vi "Get further extended drive and motor status.vi"(0 "COM port":refnum<visa-resource-name>, 7 "Drive address":T7=1 items=["0", "1", "2", "3", "4", "5", "6", "7", "8", "9", "10", "11", "12", "13", "14", "15", "16", "17", "18", "19", "20", "21", "22", "23", "24", "25", "26", "27", "28", "29", "30", "31", "32", "33", "34", "35", "36", "37", "38", "39", "40", "41", "42", "43", "44", "45", "46", "47", "48", "49", "50", "51", "52", "53", "54", "55", "56", "57", "58", "59", "60", "61", "62", "63"]) -> (4 "No errors":bool, 6 "Modbus error cluster":T1={"Checksum ok"=FALSE, "Modbus exception code"=1, "Response from correct drive"=FALSE, "Comms error"={"status"=FALSE, "code"=0, "source"=""}} {"Modbus exception code" items=["None"=0, "Invalid function request"=1, "Invalid Modbus register address"=2, "Invalid / unauthorised data value"=3, "Device failure"=4, "Request accepted, wait"=5, "Drive busy"=6, "Request rejected"=7, "Memory parity error"=8, "Gateway path unavailable"=10, "Device failed to respond"=11]}, 8 "Extended drive status":T6, 10 "Motor data":T5, 15 "Further motor and drive data":T3 {"Drive fault code" items=["No fault"=0, "Brake channel overcurrent"=1, "Brake resistor overload"=2, "Drive output overcurrent"=3, "Motor thermal overload"=4, "DC bus overvoltage"=6, "DC bus undervoltage"=7, "Heatsink overtemperature"=8, "Undertemperature"=9, "Factory default parameters loaded"=10, "External trip on DI 3"=11, "Serial comms loss trip"=12, "DC bus ripple too high"=13, "Input phase loss trip"=14, "Hardware overcurrent"=15, "Heatsink thermistor fault"=16, "Internal memory fault (IO)"=17, "Analog input current lost"=18, "Internal memory fault (DSP)"=19, "User default parameters loaded"=20, "Motor PTC thermistor trip"=21, "Internal cooling fan fault"=22, "Drive internal overheat"=23, "Drive output fault"=26, "Motor stator resistance varies"=40, "Motor stator resistance too large"=41, "Motor inductance too low"=42, "Motor inductance too high"=43, "Motor parameters not convergent"=44, "Modbus comms loss fault"=50, "CAN comms loss fault"=51]})   [LabVIEW 2020]
doc: "Modbus RTU for Invertek drives. Paul Nathan 21-JUN-2022."
uses:
  ctls/Drive address.ctl
  ctls/Extended drive status bits.ctl
  ctls/Motor data.ctl
  ctls/Further motor and drive data.ctl
  ctls/Drive fault codes.ctl
  ctls/Modbus error cluster.ctl
  ctls/Exception codes.ctl
  ctls/Register.ctl
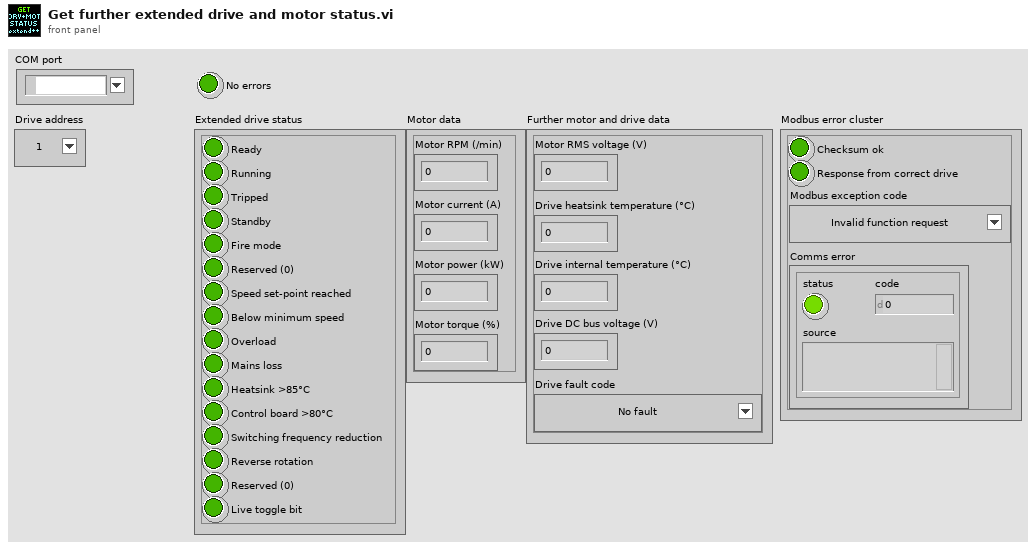
[diagram p1: front panel]
types:
  T1 = typedef "Modbus error cluster.ctl" = cluster{"Checksum ok":bool, "Modbus exception code":T2, "Response from correct drive":bool, "Comms error":errorcluster}
  T2 = typedef "Exception codes.ctl" = u8
  T3 = typedef "Further motor and drive data.ctl" = cluster{"Motor RMS voltage (V)":dbl, "Drive heatsink temperature (°C)":dbl, "Drive internal temperature (°C)":dbl, "Drive DC bus voltage (V)":dbl, "Drive fault code":T4}
  T4 = typedef "Drive fault codes.ctl" = u8
  T5 = typedef "Motor data.ctl" = cluster{"Motor RPM (/min)":dbl, "Motor current (A)":dbl, "Motor power (kW)":dbl, "Motor torque (%)":dbl}
  T6 = typedef "Extended drive status bits.ctl" = cluster{"Ready":bool, "Running":bool, "Tripped":bool, "Standby":bool, "Fire mode":bool, "Reserved (0)":bool, "Speed set-point reached":bool, "Below minimum speed":bool, "Overload":bool, "Mains loss":bool, "Heatsink >85°C":bool, "Control board >80°C":bool, "Switching frequency reduction":bool, "Reverse rotation":bool, "Reserved (0)":bool, "Live toggle bit":bool}
  T7 = typedef "Drive address.ctl" = u8
  T8 = typedef "Register.ctl" = u16
  T9 = cluster{"Boolean array[0]":bool, "Boolean array[1]":bool, "Boolean array[2]":bool, "Boolean array[3]":bool, "Boolean array[4]":bool, "Boolean array[5]":bool, "Boolean array[6]":bool, "Boolean array[7]":bool, "Boolean array[8]":bool, "Boolean array[9]":bool, "Boolean array[10]":bool, "Boolean array[11]":bool, "Boolean array[12]":bool, "Boolean array[13]":bool, "Boolean array[14]":bool, "Boolean array[15]":bool}
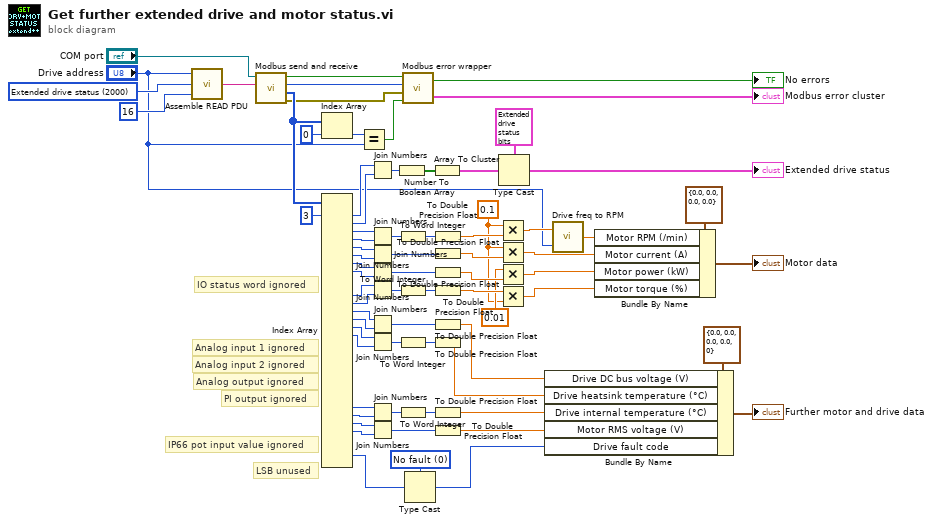
[diagram p0: block diagram]
diagram:
  w12 = T8 2000 items=["Control"=0, "RPM set-point"=4, "Drive status"=5, "Output RPM"=6, "Motor current"=7, "Motor torque"=8, "Motor power"=9, "DC bus voltage"=22, "Drive power stage temperature"=23, "kWh meter"=31, "MWh meter"=32, "Running time - hours"=33, "Running time - seconds"=34, "Internal drive temperature"=38, "Motor RMS voltage"=42, "Extended drive status"=2000] ("Register")
  w24 = T4 0 items=["No fault"=0, "Brake channel overcurrent"=1, "Brake resistor overload"=2, "Drive output overcurrent"=3, "Motor thermal overload"=4, "DC bus overvoltage"=6, "DC bus undervoltage"=7, "Heatsink overtemperature"=8, "Undertemperature"=9, "Factory default parameters loaded"=10, "External trip on DI 3"=11, "Serial comms loss trip"=12, "DC bus ripple too high"=13, "Input phase loss trip"=14, "Hardware overcurrent"=15, "Heatsink thermistor fault"=16, "Internal memory fault (IO)"=17, "Analog input current lost"=18, "Internal memory fault (DSP)"=19, "User default parameters loaded"=20, "Motor PTC thermistor trip"=21, "Internal cooling fan fault"=22, "Drive internal overheat"=23, "Drive output fault"=26, "Motor stator resistance varies"=40, "Motor stator resistance too large"=41, "Motor inductance too low"=42, "Motor inductance too high"=43, "Motor parameters not convergent"=44, "Modbus comms loss fault"=50, "CAN comms loss fault"=51] ("Drive fault code")
  w10 = 0.1 ("y")
  # "LSB unused"
  # "IP66 pot input value ignored"
  # "PI output ignored"
  # "Analog output ignored"
  # "Analog input 2 ignored"
  # "Analog input 1 ignored"
  # "IO status word ignored"
  n1 = call "Assemble READ PDU.vi"("No. of registers"=u16 16, "Register"=w12, "Drive address"="Drive address") -> ("Ser out string"=w72:string)
  n2 = call "Modbus send and receive.vi"("Modbus telegram"=w72, "COM port"="COM port") -> ("Comms error"=w2:errorcluster, "Device response"=w67:u8[], "Modbus exception code"=w1:T2, "Checksum ok"=w4:bool)  [unwired: 2 in]
  n3 = Index Array(array=w67, index=0) -> (element=w69:u8)
  n4 = Index Array(array=w67, index #1=3 ("index")) -> (element #1=w61:u8, element #2=w60:u8, element #3=w47:u8, element #4=w46:u8, element #5=w45:u8, element #6=w44:u8, element #7=w43:u8, element #8=w42:u8, element #11=w41:u8, element #12=w40:u8, element #13=w39:u8, element #14=w38:u8, element #15=w37:u8, element #16=w36:u8, element #25=w28:u8, element #26=w27:u8, element #27=w26:u8, element #28=w25:u8, element #31=w23:u8)  [unwired: 31 in, 13 out]
  n5 = Equal?(x=w69, y="Drive address") -> (x = y?=w3:bool)
  n6 = Join Numbers(hi=w61, lo=w60) -> ((hi.lo)=w59:u16)
  n7 = Join Numbers(hi=w47, lo=w46) -> ((hi.lo)=w48:u16)
  n8 = Join Numbers(hi=w45, lo=w44) -> ((hi.lo)=w51:u16)
  n9 = Join Numbers(hi=w43, lo=w42) -> ((hi.lo)=w33:u16)
  n10 = Join Numbers(hi=w41, lo=w40) -> ((hi.lo)=w35:u16)
  n11 = Join Numbers(hi=w39, lo=w38) -> ((hi.lo)=w30:u16)
  n12 = Join Numbers(hi=w37, lo=w36) -> ((hi.lo)=w31:u16)
  n13 = Join Numbers(hi=w28, lo=w27) -> ((hi.lo)=w21:u16)
  n14 = Join Numbers(hi=w26, lo=w25) -> ((hi.lo)=w22:u16)
  n15 = Number To Boolean Array(number=w59) -> (Boolean array=w65:bool[])
  n16 = To Word Integer(number=w48) -> (16bit integer=w49:i16)
  n17 = To Word Integer(number=w35) -> (16bit integer=w34:i16)
  n18 = To Word Integer(number=w31) -> (16bit integer=w32:i16)
  n19 = To Word Integer(number=w21) -> (16bit integer=w20:i16)
  n20 = call "Modbus error wrapper.vi"("Response from correct drive"=w3, "Comms error"=w2, "Modbus exception code"=w1, "Checksum ok"=w4) -> ("Modbus error cluster"=→"Modbus error cluster":T1, "No errors"=→"No errors":bool)
  n21 = Type Cast(type=w24, x=w23) -> (*(type *) &x=w13:T4)
  n22 = Array To Cluster(array=w65) -> (cluster=w64:T9)
  n23 = To Double Precision Float(number=w49) -> (double precision float=w52:dbl)
  n24 = To Double Precision Float(number=w51) -> (double precision float=w53:dbl)
  n25 = To Double Precision Float(number=w33) -> (double precision float=w54:dbl)
  n26 = To Double Precision Float(number=w34) -> (double precision float=w55:dbl)
  n27 = To Double Precision Float(number=w30) -> (double precision float=w17:dbl)
  n28 = To Double Precision Float(number=w32) -> (double precision float=w16:dbl)
  n29 = To Double Precision Float(number=w20) -> (double precision float=w15:dbl)
  n30 = To Double Precision Float(number=w22) -> (double precision float=w14:dbl)
  n31 = Multiply(x=w10, y=w52) -> (x*y=w9:dbl)
  n32 = Multiply(x=w10, y=w53) -> (x*y=w56:dbl)
  n33 = Multiply(x=0.01 ("y"), y=w54) -> (x*y=w57:dbl)
  n34 = Multiply(x=w55, y=w10) -> (x*y=w58:dbl)
  n35 = Type Cast(type=T6 {"Ready"=FALSE, "Running"=FALSE, "Tripped"=FALSE, "Standby"=FALSE, "Fire mode"=FALSE, "Reserved (0)"=FALSE, "Speed set-point reached"=FALSE, "Below minimum speed"=FALSE, "Overload"=FALSE, "Mains loss"=FALSE, "Heatsink >85°C"=FALSE, "Control board >80°C"=FALSE, "Switching frequency reduction"=FALSE, "Reverse rotation"=FALSE, "Reserved (0)"=FALSE, "Live toggle bit"=FALSE} ("Extended drive status bits"), x=w64) -> (*(type *) &x=→"Extended drive status":T6)
  n36 = Bundle By Name(cluster=T3 {"Motor RMS voltage (V)"=0.0, "Drive heatsink temperature (°C)"=0.0, "Drive internal temperature (°C)"=0.0, "Drive DC bus voltage (V)"=0.0, "Drive fault code"=0} ("Further motor and drive data"), "Drive DC bus voltage (V)"=w17, "Drive heatsink temperature (°C)"=w16, "Drive internal temperature (°C)"=w15, "Motor RMS voltage (V)"=w14, "Drive fault code"=w13) -> (→"Further motor and drive data":T3)
  n37 = call "Drive freq to RPM.vi"("Drive address"="Drive address", "Drive output f (Hz)"=w9) -> ("Motor RPM (/min)"=w8:dbl)
  n38 = Bundle By Name(cluster=T5 {"Motor RPM (/min)"=0.0, "Motor current (A)"=0.0, "Motor power (kW)"=0.0, "Motor torque (%)"=0.0} ("Motor stats"), "Motor RPM (/min)"=w8, "Motor current (A)"=w56, "Motor power (kW)"=w57, "Motor torque (%)"=w58) -> (→"Motor data":T5)
